vi "Read Holding Register.vi"(8 "error in (no error)":errorcluster, 9 "number of inputs":u16, 10 "starting address":u16, 11 "Modbus TCP in":refnum<class "Modbus TCP.lvclass">) -> (0 "error out":errorcluster, 2 "register values":u16[](array[numeric]), 3 "Modbus TCP out":refnum<class "Modbus TCP.lvclass">)   [LabVIEW 2023, in "HardwareAbstractionLayer_LVOOP.lvlib" / "Modbus TCP.lvclass"]
uses:
  Modbus TCP.lvclass
  Modbus TCP.lvclass/Modbus TCP.ctl
  <vilib>/NI/Modbus Library/API/Master/Modbus Master.lvclass
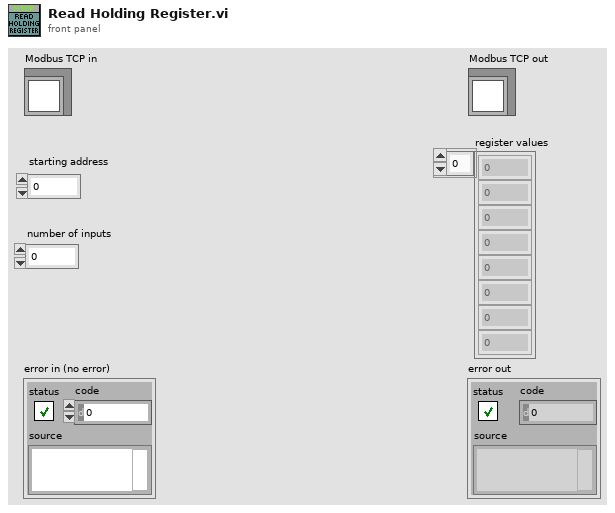
[diagram p1: front panel]
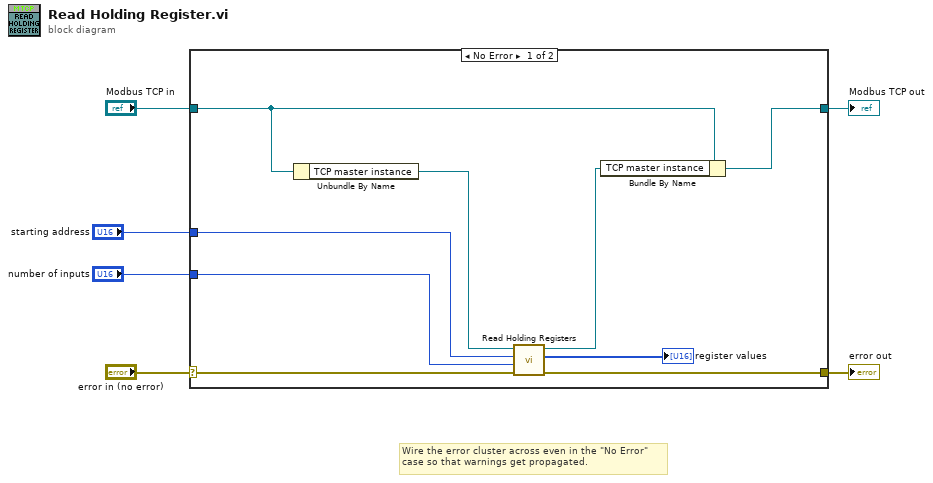
[diagram p0: block diagram]
diagram:
  # "Wire the error cluster across even in the \"No Error\"\ncase so that warnings get propagated."
  n1 = case shown="No Error" "error in (no error)" {
    selector: "error in (no error)" -> [w14 w17]
    tunnel: [w13 w17] -> w5
    tunnel: [w11 w16] -> w3
    tunnel: "Modbus TCP in" -> [w12 w16]
    tunnel: "starting address" -> [w9 _]
    tunnel: "number of inputs" -> [w8 _]
    frame No Error {
      n2 = Unbundle By Name(w12) -> ("TCP master instance"=w15:refnum<class "Modbus Master.lvclass">)
      n3 = call-dynamic "Read Holding Registers.vi"("error in"=w14, "number of inputs"=w8, "starting address"=w9, "Modbus master in"=w15) -> ("error out"=w13:errorcluster, "register values"=→"register values":u16[], "Modbus master out"=w10:refnum<class "Modbus Master.lvclass">)  [unwired: 5 in]
      n4 = Bundle By Name(cluster=w12, "TCP master instance"=w10) -> (w11:refnum<class "Modbus TCP.lvclass">)
    }
    frame Error {
    }
  }
  "error out" <- w5
  "Modbus TCP out" <- w3
